vi "3_1.vi"() -> ()   [LabVIEW 2023]
panel:
  in  "stop":bool
  out "DI Lines":bool[](array[boolean])
  out "U8 Data":u8 format="%x"
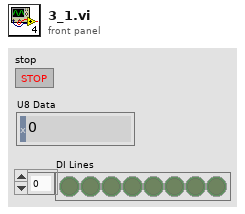
[diagram p1: front panel]
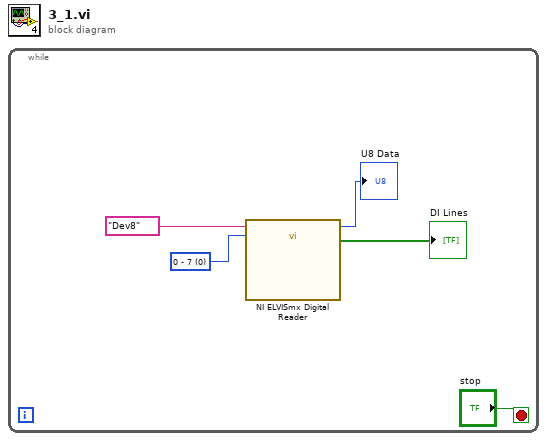
[diagram p0: block diagram]
diagram:
  n1 = while {
    stop <- "stop" stop-if-true
    w2 = u16 0 items=["0 - 7", "8 - 15", "16 - 23"] ("Lines to Read")
    n2 = call "NI ELVISmx Digital Reader"("Device Name"=tag "Dev8", "Lines to Read"=w2) -> ("U8 Data"=→"U8 Data":u8, "DI Lines"=→"DI Lines":bool[])  [unwired: 23 in, 1 out]
  }
